vi "Find Remote Terminal.vi"(8 "error in":errorcluster, 10 "terminal address":T1, 11 "port in":T2 format="%.0x") -> (0 "error out":errorcluster, 2 "remote terminal":T2 format="%.0x", 3 "port out":T2 format="%.0x", 4 "found?":bool)   [LabVIEW 2020, in "AIM MIL-STD-1553 Scripting.lvlib"]
doc: "Within the specified <b>port in</b>, searches for an instance <b>terminal address</b>. If a match is found, returns the matching <b>terminal address</b> reference. If no match is found, the returned reference is invalid and <b>found?</b> equals False."
uses:
  AIM MIL-STD-1553 Scripting.lvlib
  <vilib>/NI VeriStand/Custom Device API/Custom Device Item Ref.ctl
  Shared/Address.ctl
  <vilib>/NI VeriStand/Custom Device API/Custom Device API.lvlib
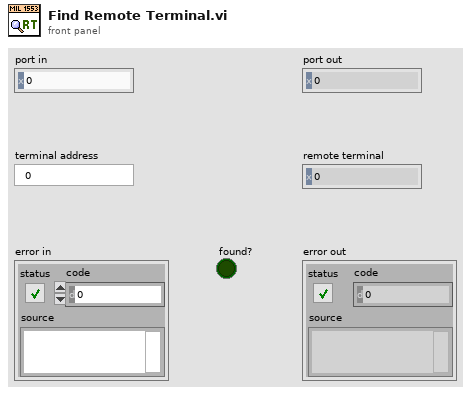
[diagram p1: front panel]
types:
  T1 = typedef "Address.ctl" = u16
  T2 = typedef "Custom Device API.lvlib/Custom Device Item Ref.ctl" = u64
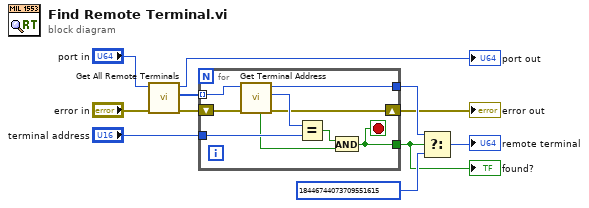
[diagram p0: block diagram]
diagram:
  n1 = call "Get All Remote Terminals.vi"("error in"="error in", "port in"="port in") -> ("error out"=w6:errorcluster, "remote terminals"=w3:T2[], "port out"=→"port out":T2)  [unwired: 7 in]
  n2 = for {
    tunnel: w3 -> [w20] mode=indexing
    tunnel: "terminal address" -> [w19]
    tunnel: [w13] -> w11
    tunnel: [w12] -> w2
    shift-right: [w14] -> w5
    shift-left: w6 -> [w15]
    stop <- w12 stop-if-true
    n3 = call "Get Terminal Address.vi"("error in"=w15, "remote terminal in"=w20) -> ("error out"=w14:errorcluster, "terminal address"=w18:T1, "remote terminal out"=w13:T2, "found?"=w17:bool)  [unwired: 6 in]
    n4 = Equal?(x=w18, y=w19) -> (x = y?=w16:bool)
    n5 = And(x=w16, y=w17) -> (x .and. y?=w12:bool)
  }
  "error out" <- w5
  "found?" <- w2
  n6 = Select(t=w11, s=w2, f=T2 18446744073709551615 ("Invalid Ref")) -> (s? t:f=→"remote terminal":T2)
